vi "FEA_Model_Intialize.vi"(8 "error in (no error)":errorcluster, 11 "FEA_Model in":refnum<class "FEA_Model.lvclass">) -> (0 "error out":errorcluster, 3 "FEA_Model out":refnum<class "FEA_Model.lvclass">)   [LabVIEW 2021, in "FEA_Model.lvclass"]
uses:
  FEA_Model.lvclass
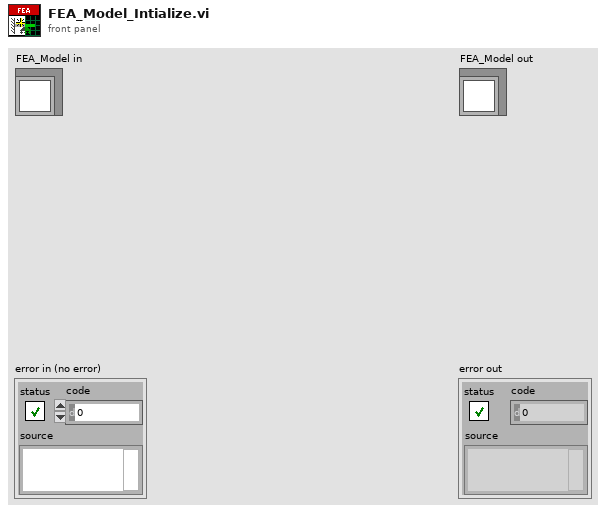
[diagram p1: front panel]
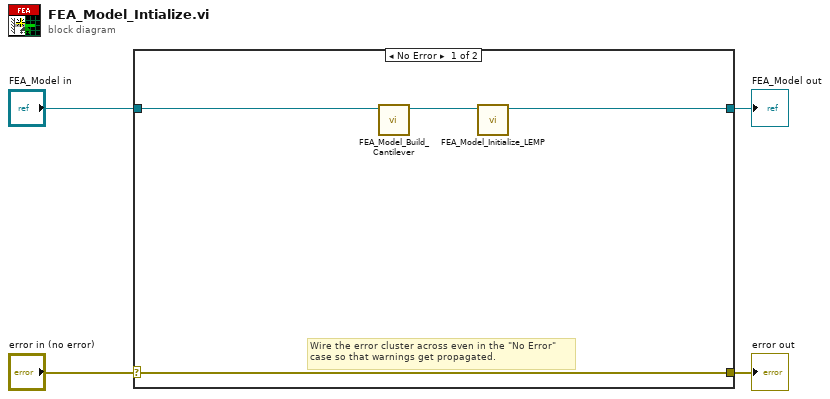
[diagram p0: block diagram]
diagram:
  n1 = case shown="No Error" "error in (no error)" {
    selector: "error in (no error)" -> [w8 w10]
    tunnel: [w8 w10] -> w3
    tunnel: [w5 w9] -> w1
    tunnel: "FEA_Model in" -> [w7 w9]
    frame No Error {
      # "Wire the error cluster across even in the \"No Error\"\ncase so that warnings get propagated."
      n2 = call "FEA_Model_Build_Cantilever.vi"("FEA_Model in"=w7) -> ("FEA_Model out"=w6:refnum<class "FEA_Model.lvclass">)  [unwired: 10 in]
      n3 = call "FEA_Model_Initialize_LEMP.vi"("FEA_Model in"=w6) -> ("FEA_Model out"=w5:refnum<class "FEA_Model.lvclass">)  [unwired: 10 in]
    }
    frame Error {
    }
  }
  "error out" <- w3
  "FEA_Model out" <- w1
